vi "PDF_Interface_PDF Protokoll T90.vi"(8 "error in (no error)":errorcluster caption="Fehler (Eingang, kein Fehler)", 10 "SVGraph Referenz":refnum<vi>, 11 "Save PDF File Path":path) -> (0 "error out":errorcluster caption="Fehler (Ausgang)")   [LabVIEW 2020, in "T90.lvlib"]
uses:
  T90.lvlib
  Zustand Auswahl.ctl
  Sprachverwaltung/FGV Aktion Tabelle zerlegen.ctl
  Aktion FGV T90.ctl
  Seiten/Gaszuordnung AO/FGV Gaszuordnung Grenzen&Einheit Aktion.ctl
  Seiten/FT-IR/FGV FT-IR Gasliste Aktionen.ctl
  PDF_Interface/PDF Protokoll Standard Kopf Optionen.ctl
  Visualisierungs Elemente/Auswahlfeld.ctl
  PDF_Interface/PDF Protokoll Standard Kopf Gasflasche Auswahl.ctl
  Seiten/System Einstellungen V2/Aktion FGV Gasbottledefinition.ctl
  Seiten/Anlagengrenzwerte/FGV Anlagengrenzwerte Aktionen.ctl
  <vilib>/Simplicity AI/SAI_PDF_API/Classes/Context/Controls/SAI_PDF_PDF Details.ctl
  PDF_Interface/PDF Interface Helper/PDFContentType.ctl
  PDF_Interface/PDF Interface Helper/PDFTableContentType.ctl
  PDF_Interface/PDF Interface Helper/PDFResults.ctl
  PDF_Interface/PDF Interface Helper/PDFResultPictures.ctl
  PDF_Interface/PDF Interface Helper/PDFCommentPosition.ctl
  PDF_Interface/PDF Interface Helper/PDFPageBreak.ctl
  PDF_Interface/PDF Interface Helper/PDFTablePictures.ctl
  PDF_Interface/PDF Interface Helper/PDFBemerkung.ctl
  <vilib>/Simplicity AI/SAI_PDF_API/Classes/Context/Controls/SAI_PDF_Text Align.ctl
  <vilib>/Simplicity AI/SAI_PDF_API/Classes/Context/Controls/SAI_PDF_Font.ctl
  <vilib>/Simplicity AI/SAI_PDF_API/Classes/Context/Controls/SAI_PDF_Font Encoding.ctl
  PDF_Interface/PDF Interface Helper/PDFGraph.ctl
  Allgemein/allgemeine Sub-VIs.lvlib
  Seiten/FT-IR/FT-IR.lvlib
  Seiten/Gaszuordnung AO/Gaszuordnung AO.lvlib
  Sprachverwaltung/Sprachverwaltung.lvlib
  PDF_Interface/PDF Interface.lvlib
  <vilib>/Simplicity AI/SAI_PDF_API/Classes/Context/Context.lvclass
  PDF_Interface/PDF Interface Helper/PDF Interface Helper.lvlib
  Seiten/Anlagengrenzwerte/Anlagengrenzwerte.lvlib
  Linearisierung V2/Protokoll/Protokoll.lvlib
  Seiten/System Einstellungen V2/System Einstellungen V2.lvlib
panel:
  out "Ergebnis":string caption="Auswertung:"
  out "T90 3":waveform(sgl)(graph) caption="T90"
  out "T90 2":waveform(sgl)(graph) caption="T90"
  out "Abschaltzeit":string caption="Abschaltzeit:"
  out "Rise Time:":string caption="T10 - T90 (Rise Time):"
  out "T10":string caption="T10 (Delay Time):"
  out "T50":string caption="T50 (Response Time):"
  out "T90":string caption="T90 (Response Time):"
  out "Einheit":string
  out "Konzentration:":string
  out "Komponente:":string
  out "Durchfluss FT-IR:":string caption="Fluss FTIR:"
  out "Abweichung:":string caption="Abweichung %:"
  out "Modus:":string
  in  "Modus: Ring":T1=1 caption="Modus:" items=["Cal Gas", "Entnahmestelle"]
  out "T90":waveform(sgl)(graph)
  # "T90 Test"
  # "IAG-Industrie Automatisierungsgeschellschaft m.b.H.    l  Industriestraße 2    l    2722Weikersdorf     )+43262221734 7+43262221734655"
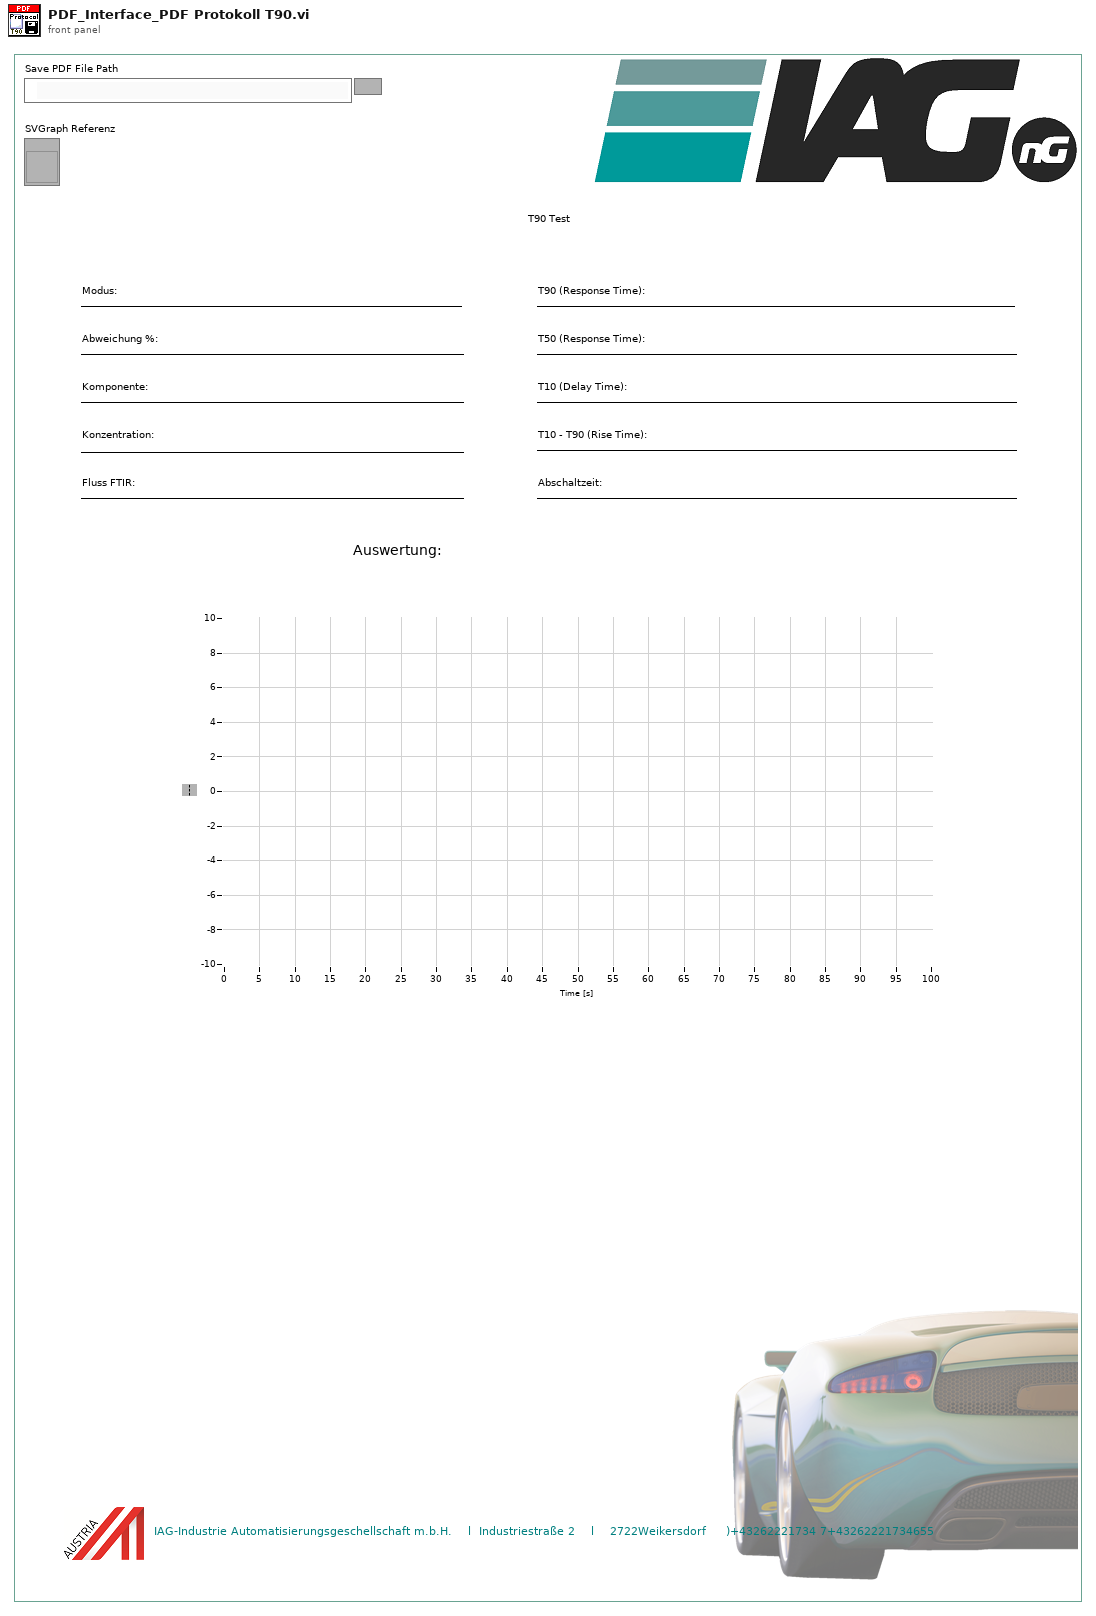
[diagram p1: front panel]
types:
  T1 = typedef "T90.lvlib/Zustand Auswahl.ctl" = u16
  T2 = typedef "Sprachverwaltung.lvlib/FGV Aktion Tabelle zerlegen.ctl" = enum16{"laden", "vereinzeln", "speichern"}
  T3 = typedef "System Einstellungen V2.lvlib/Aktion FGV Gasbottledefinition.ctl" = enum16{"lesen", "schreiben", "löschen", "laden", "speichern", "exportieren", "importieren"}
  T4 = typedef "PDF Interface.lvlib/PDF Protokoll Standard Kopf Gasflasche Auswahl.ctl" = cluster{"Gasflaschen Name":string, "Gasflaschen Nummer":string, "Gasnummer Index":i32}
  T5 = typedef "Auswahlfeld.ctl" = u16
  T6 = typedef "PDF Interface.lvlib/PDF Protokoll Standard Kopf Optionen.ctl" = cluster{"Analysator":bool, "FT-IR Rezept":bool, "Gasteiler":bool, "Gas Komponente":bool, "Gas Flasche":bool, "LIN Protokoll":bool, "Operator":bool}
  T7 = typedef "FT-IR.lvlib/FGV FT-IR Gasliste Aktionen.ctl" = enum16{"lesen", "Gasliste FT-IR", "Gasliste ausgelesen", "laden", "speichern", "löschen"}
  T8 = typedef "Gaszuordnung AO.lvlib/FGV Gaszuordnung Grenzen&Einheit Aktion.ctl" = enum16{"Lesen", "Schreiben Min", "Schreiben Max", "Laden", "Speichern"}
  T9 = typedef "T90.lvlib/Aktion FGV T90.ctl" = enum16{"lesen", "schreiben", "laden", "speichern", "T90 aktiv", "T90 Entnahme aktiv", "Overflow Leak", "Pfad", "Zustand", "max. Responsetime"}
  T10 = typedef "Anlagengrenzwerte.lvlib/FGV Anlagengrenzwerte Aktionen.ctl" = enum16{"Lesen", "Grenzwerte schreiben"}
  T11 = typedef "PDF Interface.lvlib/PDF Interface Helper.lvlib/PDFBemerkung.ctl" = cluster{"Bemerkung Text":string, "Align (Left)":T12, "Add Line Feeds (F:No)":bool, "Font":T13}
  T12 = typedef "SAI_PDF_Toolkit.lvlib/Context.lvclass/SAI_PDF_Text Align.ctl" = i32
  T13 = typedef "SAI_PDF_Toolkit.lvlib/Context.lvclass/SAI_PDF_Font.ctl" = cluster{"Font":string, "Size":i32, "Colour":u32, "Bold":bool, "Italic":bool, "Underline":bool, "Strikethrough":bool, "Font Encoding":T14}
  T14 = typedef "SAI_PDF_Toolkit.lvlib/Context.lvclass/SAI_PDF_Font Encoding.ctl" = enum16{"Cp1252, WinANSI", "IdentityH", "IdentityV", "Cp1250", "Cp1257", "MacRoman"}
  T15 = typedef "PDF Interface.lvlib/PDF Interface Helper.lvlib/PDFResults.ctl" = cluster{"Results":cluster{"Result Text":string, "Result":bool}[], "ResultPictures":T16, "use Pictures":bool, "Image Scale (%)":sgl, "Autoscale? (T)":bool, "Horizontal Align":i32, "Position":i32}
  T16 = typedef "PDF Interface.lvlib/PDF Interface Helper.lvlib/PDFResultPictures.ctl" = cluster{"Yes Ctl Refnum":refnum<vi>, "No Ctl Refnum":refnum<vi>}
  T17 = typedef "PDF Interface.lvlib/PDF Interface Helper.lvlib/PDFTableContentType.ctl" = cluster{"TableHeader":string[], "Table":string[][], "Relative Column Widths (%)":sgl[], "Results":T15, "PositionBemerkung":T18, "PageBreak":T19, "TablePictures":T20, "Horizontal Align":i32}
  T18 = typedef "PDF Interface.lvlib/PDF Interface Helper.lvlib/PDFCommentPosition.ctl" = enum16{"before", "after"}
  T19 = typedef "PDF Interface.lvlib/PDF Interface Helper.lvlib/PDFPageBreak.ctl" = enum16{"none", "before", "after", "after comment"}
  T20 = typedef "PDF Interface.lvlib/PDF Interface Helper.lvlib/PDFTablePictures.ctl" = cluster{"Ctl Refnum In":refnum<vi>[], "RowOrColumn":enum16{"Row", "Column"}, "IndexToInsert":u16, "Image Scale (%)":sgl[], "Autoscale? (T)":bool[], "Horizontal Align":i32}
  T21 = typedef "PDF Interface.lvlib/PDF Interface Helper.lvlib/PDFGraph.ctl" = cluster{"GraphCtl Refnum":refnum<vi>, "Wrap Text (F:No)":bool, "Hide Grid (F:No)":bool, "Scale (100%)":sgl, "Align (Left)":T12, "PositionBemerkung":T18, "PageBreak":T19}
  T22 = typedef "PDF Interface.lvlib/PDF Interface Helper.lvlib/PDFContentType.ctl" = cluster{"Titel":string, "Header Table":string[][], "Table Array":T17[], "Bemerkungen":T11[]}
  T23 = typedef "SAI_PDF_Toolkit.lvlib/Context.lvclass/SAI_PDF_PDF Details.ctl" = cluster{"Title":string, "Subject":string, "Keywords":string, "Author":string, "Creator":string}
  T24 = cluster{"Header Footer Text Cluster":cluster{"Header Text":string, "Footer Text":string, "Time":string, "Page Number":string}, "PDF Details":T23}
  T25 = typedef "System Einstellungen V2.lvlib/Gasflasche gesamt.ctl" = cluster{"Gasflasche":T26, "Trägergas":T27, "Komponenten":T28[]}
  T26 = typedef "System Einstellungen V2.lvlib/Gasflasche.ctl" = cluster{"Gasname für die Auswahl":string, "Chargennummer":string, "Ablaufdatum":timestamp}
  T27 = typedef "System Einstellungen V2.lvlib/Traegergas.ctl" = string
  T28 = typedef "System Einstellungen V2.lvlib/Gasflaschenkomponente.ctl" = cluster{"Gasauswahl":string, "Konzentration IST":dbl, "Einheit":string, "Genauigkeit":dbl}
  T29 = typedef "T90.lvlib/T90 Gas Konfig.ctl" = cluster{"Gasflasche":T30, "Konfig Gasflasche":T31, "Auswahl":T5, "Sollwert":T32, "Abweichung":T32, "max. Responsetime":T32, "Modus:":T1, "Abschaltzeit":T32, "Stabilisierungszeit":T32, "Bearbeiter":string}
  T30 = typedef "System Einstellungen V2.lvlib/Gasflasche Auswahl.ctl" = u16
  T31 = typedef "System Einstellungen V2.lvlib/Konfig Gasflasche.ctl" = bool
  T32 = typedef "Zahlen-Eingabefeld.ctl" = sgl
  T33 = typedef "Anlagengrenzwerte.lvlib/Anlagen-Grenzwerte Anzeige.ctl" = cluster{"Eingangsdruck FT-IR:":T34, "Durchfluss FT-IR:":T34, "Durchfluss CalGas:":T34, "Druck Ausgang:":T34, "Druck Kalter Block:":T34, "Heizleitungen intern:":T34, "Heizleitung zu FT-IR:":T34, "Heizung Filterblock:":T34, "Heizung Pumpe:":T34, "Heizleitung Extern SP1:":T34, "Heizleitung Extern SP2:":T34, "FT-IR Heizung Messzelle:":T34, "Schaltschranktemperatur:":T34, "Gaskühler:":T34}
  T34 = typedef "Anlagengrenzwerte.lvlib/Anlagen-Parameter Anzeige.ctl" = cluster{"Sollwert":sgl, "Warn-Min":sgl, "Warn-Max":sgl, "Abschalt-Min":sgl, "Abschalt-Max":sgl, "Regler":u16}
  T35 = typedef "String - Ausgabefeld.ctl" = string
  T36 = cluster{"Signalverlauf":waveform(sgl), "T90":dbl, "T50":dbl, "T10":dbl, "Rise time ":dbl, "Bestanden?":bool}
  T37 = cluster{"Header Size":i32, "Column Ratio left":sgl[]}
  T38 = cluster{"String - Ausgabefeld":T35, "Bestanden?":bool}
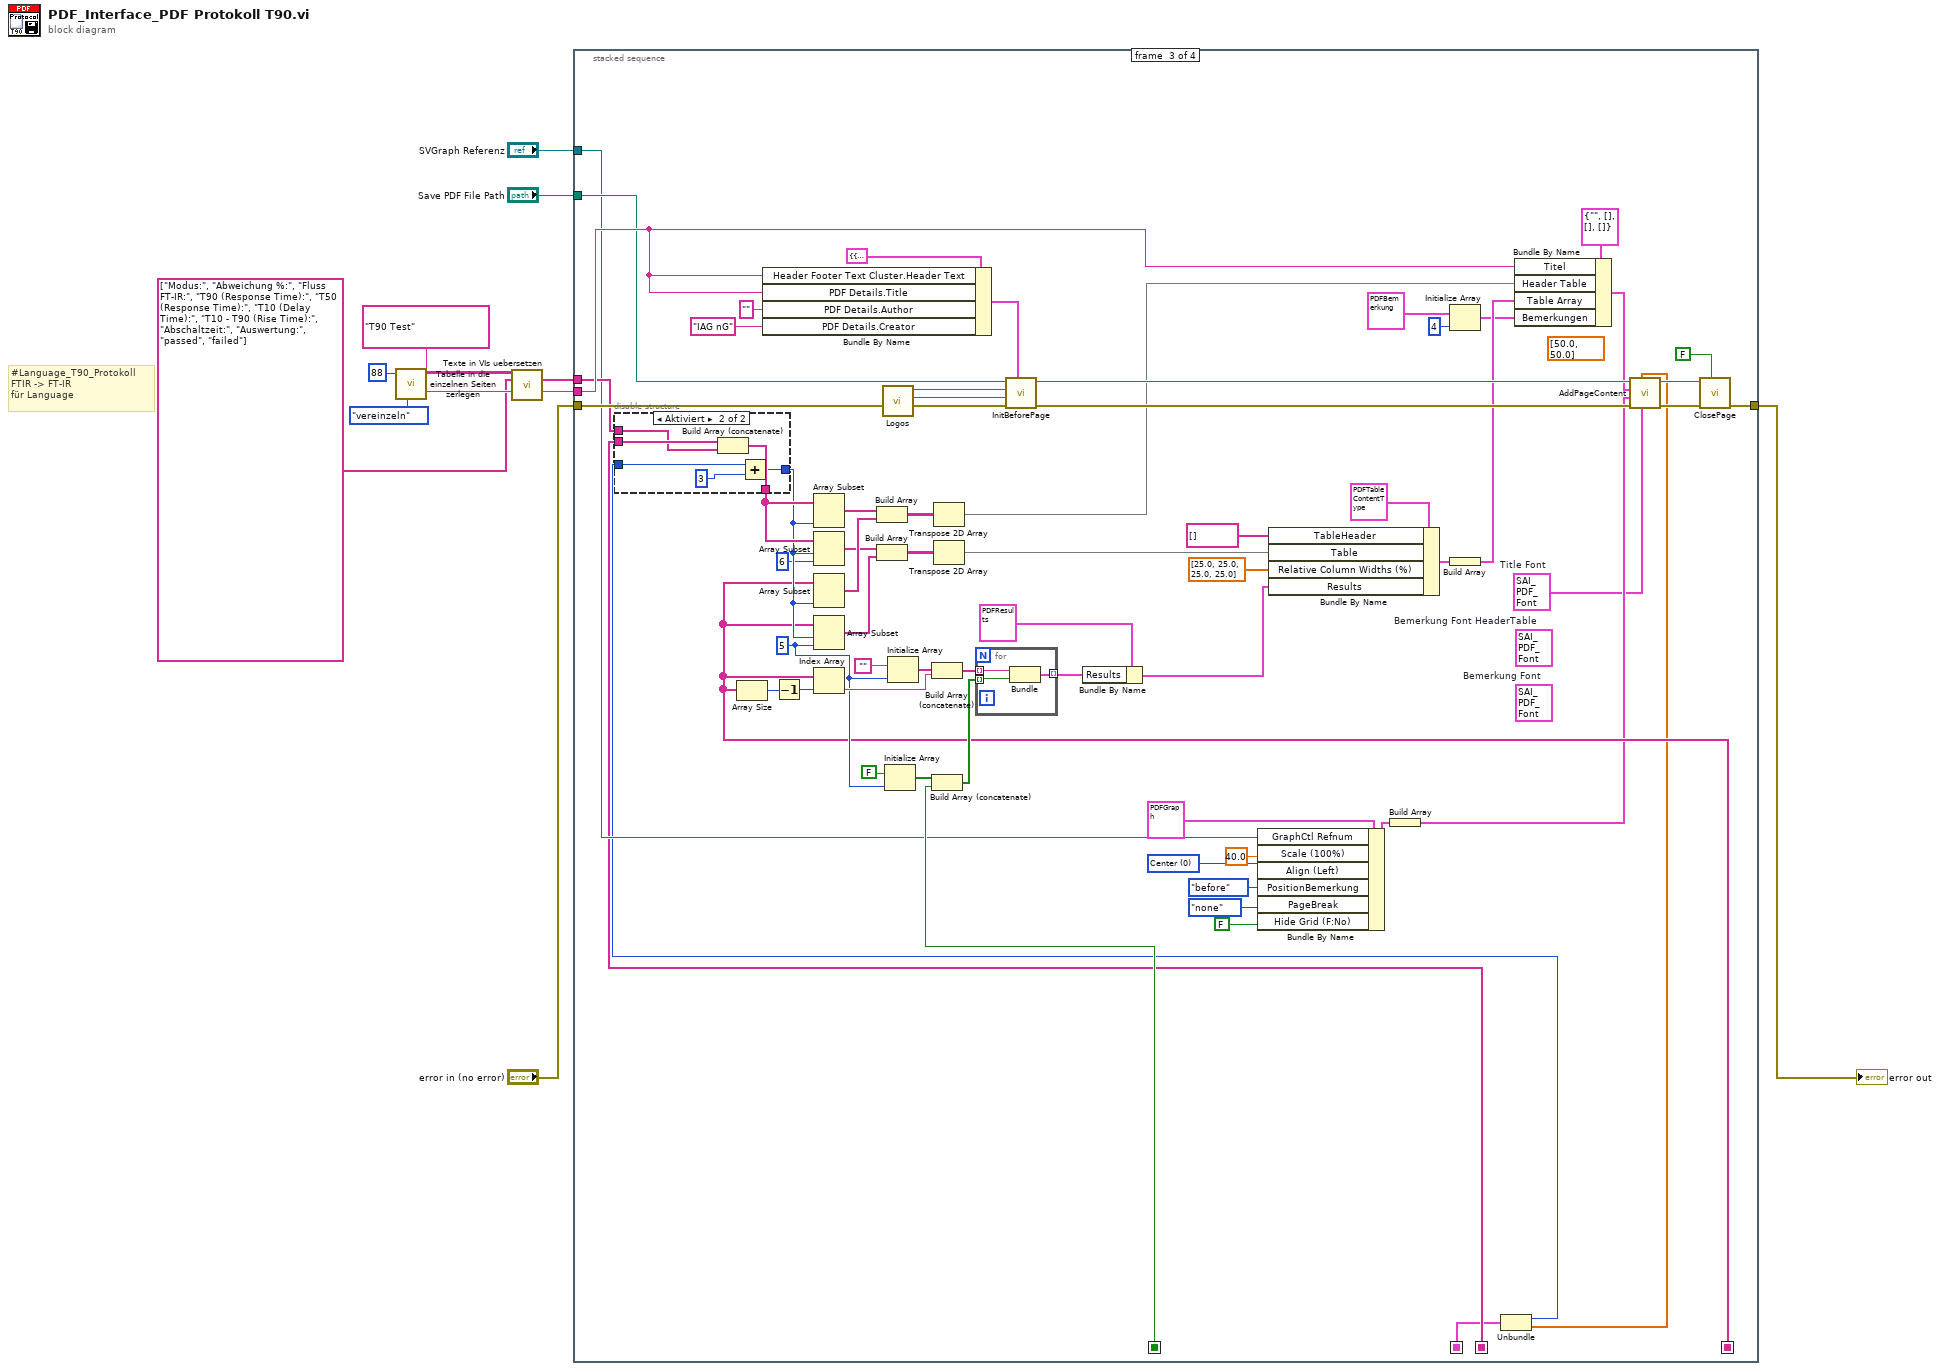
[diagram p0: block diagram]
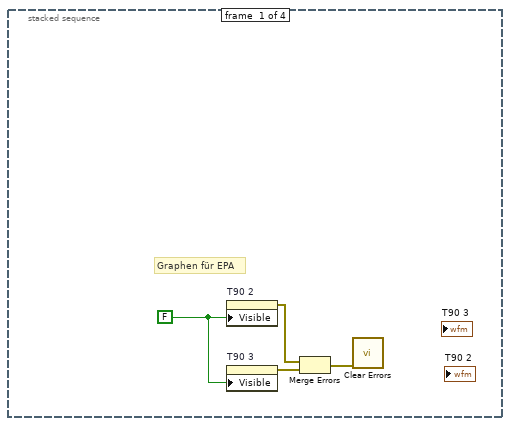
[diagram p2: hidden frame]
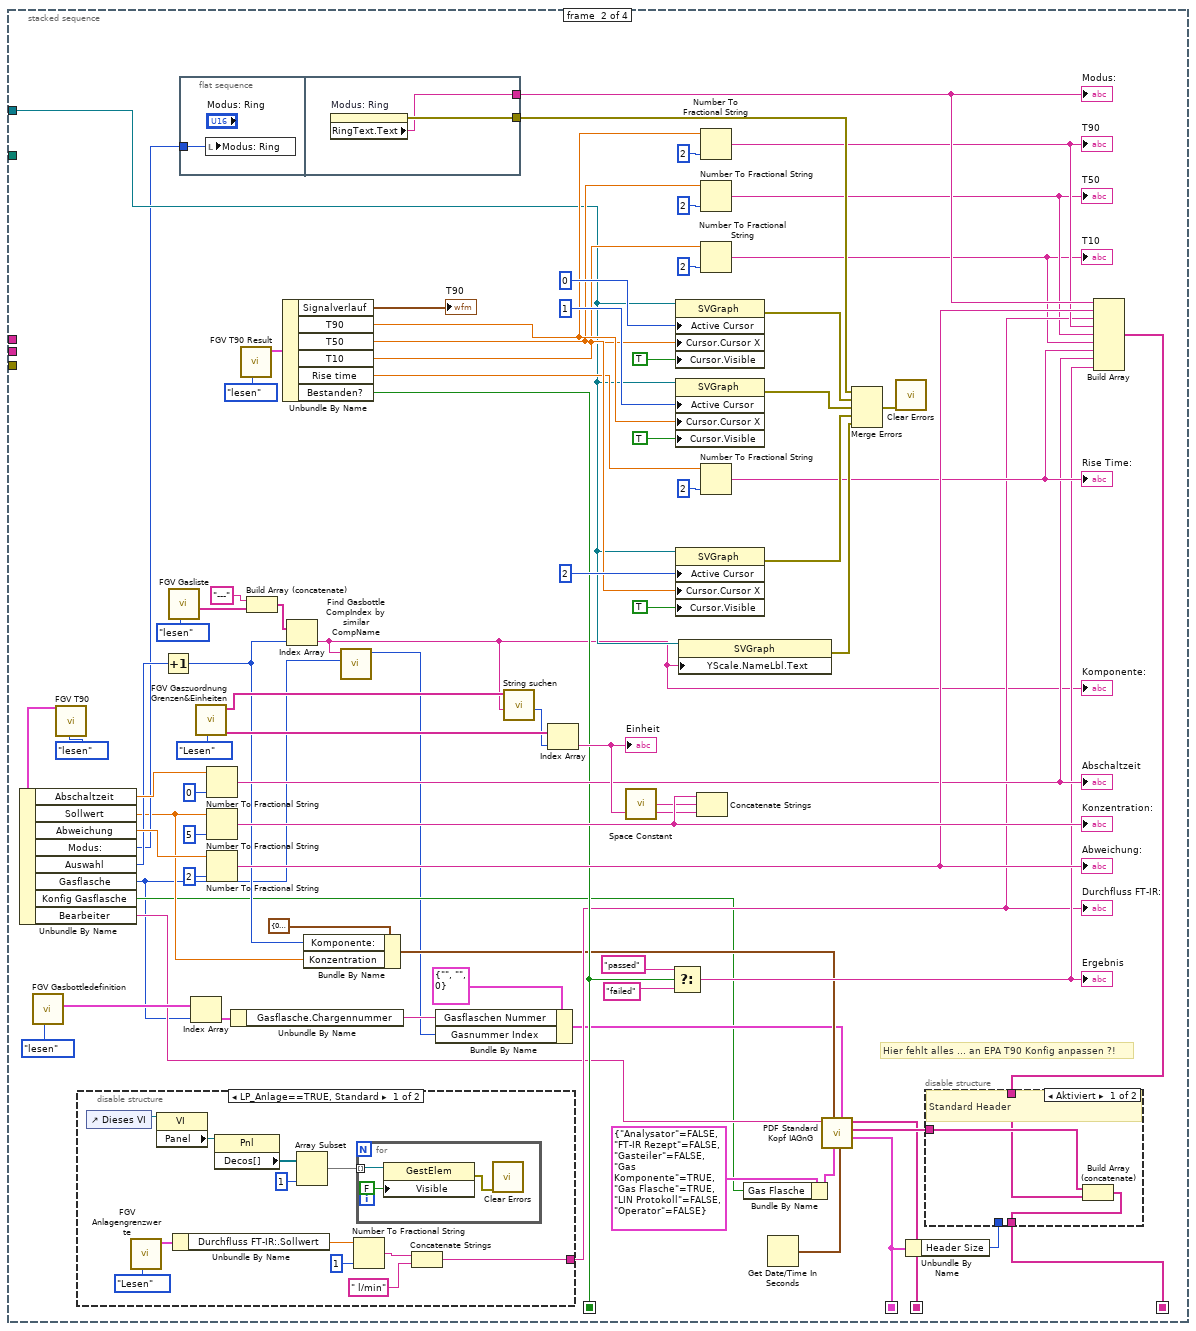
[diagram p3: hidden frame]
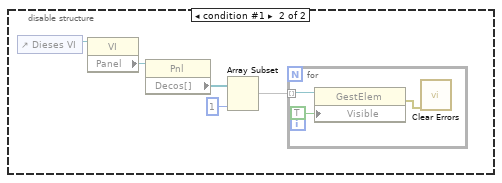
[diagram p5: hidden frame]
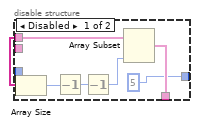
[diagram p6: hidden frame]
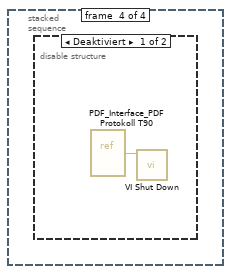
[diagram p7: hidden frame]
diagram:
  # "#Language_T90_Protokoll\nFTIR -> FT-IR \nfür Language"
  n1 = call "Tabelle in die einzelnen Seiten zerlegen.vi"("Aktion"=FGV_Aktion_Tabelle_zerlegen."vereinzeln", "Index (Seite)"=88) -> ("Sprachliste"=w9:string[][])  [unwired: 7 in, 2 out]
  n2 = call "Texte in VIs uebersetzen.vi"("Sprachliste"=w9, "String-Array zum Übersetzen"=string[] ["Modus:", "Abweichung %:", "Fluss FT-IR:", "T90 (Response Time):", "T50 (Response Time):", "T10 (Delay Time):", "T10 - T90 (Rise Time):", "Abschaltzeit:", "Auswertung:", "passed", "failed"], "String zum Übersetzen"="T90 Test") -> ("String-Array zum Übersetzen"=w5:string[], "String zum Übersetzen"=w6:string)  [unwired: 8 in, 3 out]
  n3 = stacked-sequence {
    seq-local: [_ w36 _ _] -> [_ _ w150 _]
    seq-local: [_ w44 _ _] -> [_ _ w149 _]
    seq-local: [_ w27 _ _] -> [_ _ w128 _]
    seq-local: [_ w34 _ _] -> [_ _ w129 _]
    tunnel: w6 -> [_ _ w153 _]
    tunnel: w5 -> [_ _ w148 _]
    tunnel: "Save PDF File Path" -> [_ _ w147 _]
    tunnel: "SVGraph Referenz" -> [_ w54 w139 _]
    tunnel: "error in (no error)" -> [_ _ w152 _]
    tunnel: [_ _ w151 _] -> w1
    frame #0 {
      w15 = FALSE
      # "Graphen für EPA"
      n4 = property on="T90 2" class="SVGraph (strikt)"("Visible"=w15) -> (error out=w13:errorcluster)  [unwired: 2 in, 1 out]
      n5 = property on="T90 3" class="SVGraph (strikt)"("Visible"=w15) -> (error out=w12:errorcluster)  [unwired: 2 in, 1 out]
      n6 = Merge Errors(w13, w12) -> (w14:errorcluster)
      n7 = call <vilib>:"Clear Errors.vi"("error in (no error)"=w14) -> ()  [unwired: 5 in, 2 out]
    }
    frame #1 {
      # "Hier fehlt alles ... an EPA T90 Konfig anpassen ?!"
      n8 = call "FGV Gasbottledefinition.vi"("Aktion"=Aktion_FGV_Gasbottledefinition."lesen") -> ("Gasflaschen Liste gesamt"=w24:T25[])  [unwired: 8 in, 2 out]
      n9 = call "FGV T90.vi"("Aktion"=Aktion_FGV_T90."lesen") -> ("Gas Konfig"=w59:T29)  [unwired: 20 in, 6 out]
      n10 = Unbundle By Name(w59) -> ("Abschaltzeit"=w58:T32, "Sollwert"=w31:T32, "Abweichung"=w57:T32, "Modus:"=w43:T1, "Auswahl"=w56:T5, "Gasflasche"=w17:T30, "Konfig Gasflasche"=w19:T31, "Bearbeiter"=w21:string)
      n11 = disable-structure shown="LP_Anlage==TRUE, Standard" {
        disable-tunnel: [w101 _] -> w42
        frame condition #0 (active) {
          n12 = control-ref of="Dieses VI"() -> (w107:refnum<vi>)
          n13 = call "FGV Anlagengrenzwerte.vi"("Aktion"=FGV_Anlagengrenzwerte_Aktionen."Lesen") -> ("Anlagen-Grenzwerte Anzeige"=w109:T33)  [unwired: 1 in, 9 out]
          n14 = property class="VI"(reference=w107) -> ("Panel"=w104:refnum<vi>)  [unwired: 1 in, 2 out]
          n15 = Unbundle By Name(w109) -> ("Durchfluss FT-IR:.Sollwert"=w108:sgl)
          n16 = property class="Pnl"(reference=w104) -> ("Decos[]"=w105:refnum<vi>[])  [unwired: 1 in, 2 out]
          n17 = Array Subset(array=w105, length=1 ("Länge")) -> (w106:refnum<vi>[])  [unwired: 1 in]
          n18 = Number To Fractional String(number=w108, precision (6)=i16 1 ("Genauigkeit (6)")) -> (F-format string=w102:string)  [unwired: 2 in]
          n19 = for {
            tunnel: w106 -> [w114] mode=indexing
            n20 = property class="GestElem"(reference=w114, "Visible"=FALSE ("Sichtbar")) -> (error out=w112:errorcluster)  [unwired: 1 in, 1 out]
            n21 = call <vilib>:"Clear Errors.vi"("error in (no error)"=w112) -> ()  [unwired: 5 in, 2 out]
          }
          n22 = Concatenate Strings(w102, " l/min" ("Einheit 2")) -> (w101:string)
        }
        frame condition #1 {
          n23 = control-ref of="Dieses VI"() -> (w119:refnum<vi>)
          n24 = property class="VI"(reference=w119) -> ("Panel"=w116:refnum<vi>)  [unwired: 1 in, 2 out]
          n25 = property class="Pnl"(reference=w116) -> ("Decos[]"=w117:refnum<vi>[])  [unwired: 1 in, 2 out]
          n26 = Array Subset(array=w117, length=1 ("Länge")) -> (w118:refnum<vi>[])  [unwired: 1 in]
          n27 = for {
            tunnel: w118 -> [w122] mode=indexing
            n28 = property class="GestElem"(reference=w122, "Visible"=TRUE ("Sichtbar")) -> (error out=w120:errorcluster)  [unwired: 1 in, 1 out]
            n29 = call <vilib>:"Clear Errors.vi"("error in (no error)"=w120) -> ()  [unwired: 5 in, 2 out]
          }
        }
      }
      "Durchfluss FT-IR:" <- w42
      n30 = Increment(x=w56) -> (x+1=w32:T5)
      n31 = call "FGV Gasliste.vi"("Aktionen"=FGV_FT-IR_Gasliste_Aktionen."lesen") -> ("Aktuelle Gasliste gesamt"=w84:T35[])  [unwired: 8 in, 2 out]
      n32 = flat-sequence {
        tunnel: w43 -> [w123]
        tunnel: [w125] -> w69
        tunnel: [w124] -> w50
        frame #0 {
          n33 = local write "Modus: Ring"(w123) -> ()
        }
        frame #1 {
          n34 = property on="Modus: Ring" class="Ring (strikt)"() -> (error out=w125:errorcluster, "RingText.Text"=w124:string)  [unwired: 2 in, 1 out]
        }
      }
      n35 = Index Array(array=w24, index=w17) -> (element=w23:T25)
      n36 = call "FGV Gaszuordnung Grenzen&Einheiten.vi"("Aktion"=FGV_Gaszuordnung_Grenzen&Einheit_Aktion."Lesen") -> ("Einheit neu"=w82:string[], "Namen neu"=w64:string[])  [unwired: 7 in, 2 out]
      n37 = Number To Fractional String(number=w58, precision (6)=i16 0 ("Genauigkeit (6)")) -> (F-format string=w46:string)  [unwired: 2 in]
      "Abschaltzeit" <- w46
      n38 = Number To Fractional String(number=w31, precision (6)=i16 5 ("Genauigkeit (6)")) -> (F-format string=w53:string)  [unwired: 2 in]
      "Konzentration:" <- w53
      n39 = Number To Fractional String(number=w57, precision (6)=i16 2 ("Genauigkeit (6)")) -> (F-format string=w49:string)  [unwired: 2 in]
      "Abweichung:" <- w49
      n40 = Unbundle By Name(w23) -> ("Gasflasche.Chargennummer"=w22:string)
      n41 = call "FGV T90 Result.vi"("Aktion"=enum16{"lesen", "schreiben"}."lesen") -> ("T90 Cluster out"=w78:T36)  [unwired: 10 in]
      n42 = Build Array (concatenate)("---", w84) -> (w85:T35[])
      n43 = Unbundle By Name(w78) -> ("Signalverlauf"=→"T90":waveform(sgl), "T90"=w73:dbl, "T50"=w72:dbl, "T10"=w71:dbl, "Rise time"=w70:dbl, "Bestanden?"=w44:bool)
      n44 = Index Array(array=w85, index=w32) -> (element=w18:T35)
      "Komponente:" <- w18
      n45 = Bundle By Name(cluster=cluster{"Komponente:":T5, "Konzentration":dbl} {"Komponente:"=0, "Konzentration"=0.0} ("Gas Komponente"), "Komponente:"=w32, "Konzentration"=w31) -> (w30:cluster{"Komponente:":T5, "Konzentration":dbl})
      n46 = call "Find Gasbottle CompIndex by similar CompName.vi"("Botle Index"=w17, "Comp Name"=w18) -> ("Gas Component Index in Bottle"=w16:i32)  [unwired: 3 in, 6 out]
      n47 = Bundle By Name(cluster=T4 {"Gasflaschen Name"="", "Gasflaschen Nummer"="", "Gasnummer Index"=0} ("Gaschflasche Cluster"), "Gasflaschen Nummer"=w22, "Gasnummer Index"=w16) -> (w28:T4)
      n48 = call "String suchen.vi"("Gasname"=w18, "Such-Namen"=w64) -> ("Index"=w63:i32)  [unwired: 8 in, 1 out]
      n49 = Index Array(array=w82, index=w63) -> (element=w51:string)
      "Einheit" <- w51
      n50 = call <vilib>:"Space Constant.vi"() -> ("String"=w52:string)
      n51 = Select(t="passed", s=w44, f="failed") -> (s? t:f=w45:string)
      "Ergebnis" <- w45
      n52 = property on="Eigenschaftsknoten" class="SVGraph"(reference=w54, "Active Cursor"=u32 0 ("Aktiver Cursor"), "Cursor.Cursor X"=w71, "Cursor.Visible"=TRUE ("Cursor.Sichtbar")) -> (error out=w68:errorcluster)  [unwired: 1 in, 1 out]
      n53 = property on="Eigenschaftsknoten" class="SVGraph"(reference=w54, "Active Cursor"=u32 1 ("Aktiver Cursor"), "Cursor.Cursor X"=w73, "Cursor.Visible"=TRUE ("Cursor.Sichtbar")) -> (error out=w67:errorcluster)  [unwired: 1 in, 1 out]
      n54 = property on="Eigenschaftsknoten" class="SVGraph"(reference=w54, "Active Cursor"=u32 2 ("Aktiver Cursor"), "Cursor.Cursor X"=w72, "Cursor.Visible"=TRUE ("Cursor.Sichtbar")) -> (error out=w66:errorcluster)  [unwired: 1 in, 1 out]
      n55 = property on="Eigenschaftsknoten" class="SVGraph"(reference=w54, "YScale.NameLbl.Text"=w18) -> (error out=w65:errorcluster)  [unwired: 1 in, 1 out]
      n56 = Concatenate Strings(w53, w52, w51) -> ()  [unwired: 1 out]
      n57 = Number To Fractional String(number=w73, precision (6)=i16 2 ("Genauigkeit (6)")) -> (F-format string=w48:string)  [unwired: 2 in]
      "T90" <- w48
      n58 = Number To Fractional String(number=w72, precision (6)=i16 2 ("Genauigkeit (6)")) -> (F-format string=w41:string)  [unwired: 2 in]
      "T50" <- w41
      n59 = Number To Fractional String(number=w71, precision (6)=i16 2 ("Genauigkeit (6)")) -> (F-format string=w40:string)  [unwired: 2 in]
      "T10" <- w40
      n60 = Number To Fractional String(number=w70, precision (6)=i16 2 ("Genauigkeit (6)")) -> (F-format string=w47:string)  [unwired: 2 in]
      "Rise Time:" <- w47
      n61 = Bundle By Name(cluster=T6 {"Analysator"=FALSE, "FT-IR Rezept"=FALSE, "Gasteiler"=FALSE, "Gas Komponente"=TRUE, "Gas Flasche"=TRUE, "LIN Protokoll"=FALSE, "Operator"=FALSE} ("Oprtionen Cluster"), "Gas Flasche"=w19) -> (w20:T6)
      n62 = Get Date/Time In Seconds() -> (seconds since 1Jan1904=w38:timestamp)
      n63 = call "PDF Standard Kopf IAGnG.vi"("Zeitstempel"=w38, "Gaschflasche Cluster"=w28, "Oprtionen Cluster"=w20, "Gas Komponente"=w30, "Bearbeiter/in"=w21) -> ("Size Cluster"=w27:T37, "Header Values"=w35:T35[], "Header Labels"=w34:string[])  [unwired: 3 in, 1 out]
      n64 = Merge Errors(w69, w68, w67, w66, w65) -> (w89:errorcluster)
      n65 = call <vilib>:"Clear Errors.vi"("error in (no error)"=w89) -> ()  [unwired: 5 in, 2 out]
      n66 = Unbundle By Name(w27) -> ("Header Size"=w26:i32)
      n67 = Build Array(w50, w49, w42, w48, w41, w40, w47, w46, w45) -> (w37:string[])
      n68 = disable-structure shown="Aktiviert" {
        disable-tunnel: w37 -> [w96 w99]
        disable-tunnel: w35 -> [w98 _]
        disable-tunnel: [w97 w99] -> w36
        disable-tunnel: w26 -> [_ _]
        frame Enabled {
          # "Standard Header"
          n69 = Build Array (concatenate)(w98, w96) -> (w97:T35[])
        }
        frame Disabled {
        }
      }
      "Modus:" <- w50
    }
    frame #2 {
      (unwired) T13 {"Font"="Arial", "Size"=12, "Colour"=16711680, "Bold"=TRUE, "Italic"=TRUE, "Underline"=FALSE, "Strikethrough"=FALSE, "Font Encoding"=enum."Cp1252, WinANSI"}  # Bemerkung Font HeaderTable
      (unwired) T13 {"Font"="Arial", "Size"=12, "Colour"=0, "Bold"=TRUE, "Italic"=TRUE, "Underline"=FALSE, "Strikethrough"=FALSE, "Font Encoding"=enum."Cp1252, WinANSI"}  # Bemerkung Font
      w135 = T13 {"Font"="Arial", "Size"=26, "Colour"=0, "Bold"=TRUE, "Italic"=FALSE, "Underline"=TRUE, "Strikethrough"=FALSE, "Font Encoding"=enum."Cp1252, WinANSI"}  # Title Font
      w141 = T12 0 items=["Center", "Justified", "Justified All", "Left", "Right"] ("Align (Left)")
      (unwired) sgl[] [50.0, 50.0] ("Column Ratio left")
      w154 = 5 ("Länge")
      n70 = Array Size(array=w150) -> (size(s)=w173:i32)
      n71 = Bundle By Name(cluster=T24 {"Header Footer Text Cluster"={"Header Text"="Protokoll XYZ", "Footer Text"="IAG nG", "Time"="<TIMESTAMP yyyy-MM-dd>", "Page Number"="Page <P> of <PT>"}, "PDF Details"={"Title"="Test PDF", "Subject"="Versa Tabasco", "Keywords"="", "Author"="RIW", "Creator"="IAG"}} ("Info"), "Header Footer Text Cluster.Header Text"=w153, "PDF Details.Title"=w153, "PDF Details.Author"="", "PDF Details.Creator"="IAG nG") -> (w181:T24)
      n72 = Decrement(x=w173) -> (x-1=w165:i32)
      n73 = Index Array(array=w150, index=w165) -> (element=w170:T35)
      n74 = call "Logos.vi"() -> ("Footer Image File Path"=w190:path, "Header Image File Path"=w191:path)  [unwired: 8 in, 2 out]
      n75 = Initialize Array(FALSE, w154) -> (w163:bool[])
      n76 = Initialize Array("", w154) -> (w171:string[])
      n77 = Build Array (concatenate)(w171, w170) -> (w162:T35[])
      n78 = Build Array (concatenate)(w163, w149) -> (w161:bool[])
      n79 = for {
        tunnel: w162 -> [w206] mode=indexing
        tunnel: w161 -> [w205] mode=indexing
        tunnel: [w204] -> w131 mode=indexing
        n80 = Bundle("String - Ausgabefeld"=w206, "Bestanden?"=w205) -> (w204:T38)  [unwired: 1 in]
      }
      n81 = call "InitBeforePage.vi"("Info"=w181, "Fehler (Eingang, kein Fehler)"=w152, "Footer Image File Path"=w190, "Header Image File Path"=w191, "Path (Dialog if Empty)"=w147) -> ("Fehler (Ausgang)"=w189:errorcluster, "Context (Ausgang)"=w188:refnum<class "Context.lvclass">)  [unwired: 5 in]
      n82 = Bundle By Name(cluster=T15 {"Results"=[], "ResultPictures"={"Yes Ctl Refnum"=refnum, "No Ctl Refnum"=refnum}, "use Pictures"=FALSE, "Image Scale (%)"=100.0, "Autoscale? (T)"=TRUE, "Horizontal Align"=3, "Position"=0} ("Results"), "Results"=w131) -> (w132:T15)
      n83 = Bundle By Name(cluster=T21 {"GraphCtl Refnum"=refnum, "Wrap Text (F:No)"=FALSE, "Hide Grid (F:No)"=FALSE, "Scale (100%)"=100.0, "Align (Left)"=0, "PositionBemerkung"=enum."before", "PageBreak"=enum."after comment"} ("Graph"), "GraphCtl Refnum"=w139, "Scale (100%)"=sgl 40.0, "Align (Left)"=w141, "PositionBemerkung"=PDFCommentPosition."before", "PageBreak"=PDFPageBreak."none", "Hide Grid (F:No)"=FALSE) -> (w145:T21)
      n84 = Build Array(w145) -> (w138:T21[])
      n85 = Initialize Array(T11 {"Bemerkung Text"="", "Align (Left)"=0, "Add Line Feeds (F:No)"=FALSE, "Font"={"Font"="Arial", "Size"=10, "Colour"=0, "Bold"=FALSE, "Italic"=FALSE, "Underline"=FALSE, "Strikethrough"=FALSE, "Font Encoding"=enum."Cp1252, WinANSI"}} ("Bemerkung"), 4 ("Dimensionsgröße")) -> (w137:T11[])
      n86 = Unbundle(w128) -> ("Header Size"=w127:i32, "Column Ratio left"=w126:sgl[])
      n87 = disable-structure shown="Aktiviert" {
        disable-tunnel: [w194 w202] -> w176
        disable-tunnel: [5 ("Länge") w199] -> w175
        disable-tunnel: w148 -> [w193 w200]
        disable-tunnel: w129 -> [_ w203]
        disable-tunnel: w127 -> [_ w201]
        frame Disabled {
          n88 = Array Size(array=w193) -> (size(s)=w197:i32)
          n89 = Decrement(x=w197) -> (x-1=w196:i32)
          n90 = Decrement(x=w196) -> (x-1=w195:i32)
          n91 = Array Subset(array=w193, length=w195) -> (w194:string[])  [unwired: 1 in]
        }
        frame Enabled {
          n92 = Build Array (concatenate)(w203, w200) -> (w202:string[])
          n93 = Add(x=w201, y=3 ("Länge")) -> (x+y=w199:i32)
        }
      }
      n94 = Array Subset(array=w176, length=w175) -> (w179:string[])  [unwired: 1 in]
      n95 = Array Subset(array=w176, index=w175, length=6 ("Länge")) -> (w168:string[])
      n96 = Array Subset(array=w150, length=w175) -> (w178:T35[])  [unwired: 1 in]
      n97 = Array Subset(array=w150, index=w175, length=w154) -> (w167:T35[])
      n98 = Build Array(w179, w178) -> (w177:T35[][])
      n99 = Build Array(w168, w167) -> (w166:T35[][])
      n100 = Transpose 2D Array(2D array=w177) -> (transposed array=w156:T35[][])
      n101 = Transpose 2D Array(2D array=w166) -> (transposed array=w155:T35[][])
      n102 = Bundle By Name(cluster=T17 {"TableHeader"=[], "Table"=[], "Relative Column Widths (%)"=[], "Results"={"Results"=[], "ResultPictures"={"Yes Ctl Refnum"=refnum, "No Ctl Refnum"=refnum}, "use Pictures"=FALSE, "Image Scale (%)"=0.0, "Autoscale? (T)"=FALSE, "Horizontal Align"=0, "Position"=0}, "PositionBemerkung"=enum."before", "PageBreak"=enum."none", "TablePictures"={"Ctl Refnum In"=[], "RowOrColumn"=enum."Row", "IndexToInsert"=0, "Image Scale (%)"=[], "Autoscale? (T)"=[], "Horizontal Align"=0}, "Horizontal Align"=0} ("Table Array"), "TableHeader"=string[] [], "Table"=w155, "Relative Column Widths (%)"=sgl[] [25.0, 25.0, 25.0, 25.0], "Results"=w132) -> (w159:T17)
      n103 = Build Array(w159) -> (w158:T17[])
      n104 = Bundle By Name(cluster=T22 {"Titel"="", "Header Table"=[], "Table Array"=[], "Bemerkungen"=[]} ("Content"), "Titel"=w153, "Header Table"=w156, "Table Array"=w158, "Bemerkungen"=w137) -> (w157:T22)
      n105 = call "AddPageContent.vi"("Title Font"=w135, "Column Ratio left"=w126, "error in"=w189, "Graph Array"=w138, "Content"=w157, "Context (Eingang)"=w188) -> ("error out"=w187:errorcluster, "Context (Ausgang)"=w186:refnum<class "Context.lvclass">)  [unwired: 4 in]
      n106 = call "ClosePage.vi"("popup viewer"=FALSE, "Fehler (Eingang, kein Fehler)"=w187, "Context (Eingang)"=w186) -> ("Fehler (Ausgang)"=w151:errorcluster)  [unwired: 8 in]
    }
    frame #3 {
      n107 = disable-structure shown="Deaktiviert" {
        frame Disabled {
          n108 = vi-ref "PDF_Interface_PDF Protokoll T90.vi"() -> (w207:refnum<vi>)
          n109 = call "VI Shut Down.vi"("VI Referenz"=w207) -> ()  [unwired: 11 in]
        }
        frame Enabled {
        }
      }
    }
  }
  "error out" <- w1
